vi "DefaultBaseDirectory.vi"(11 "base directory in":path) -> (3 "base directory":path)   [LabVIEW 2017, in "GlobalConfiguration.lvlib"]
uses:
  <vilib>/addons/InsightCM/Utilities/GlobalConfiguration/GlobalConfiguration.lvlib
panel:
  # "Note: Set this before anything else runs"
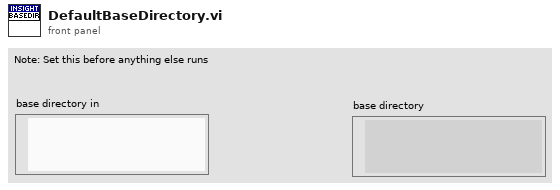
[diagram p1: front panel]
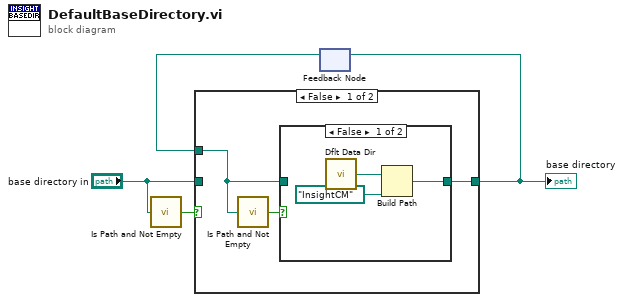
[diagram p0: block diagram]
diagram:
  n1 = call <vilib>:"Is Path and Not Empty.vi"("path"="base directory in") -> ("Is Path and Not Empty?"=w4:bool)  [unwired: 4 in]
  n2 = feedback #1() -> (w2:path)  [unwired: 1 in]
  n3 = case shown="False" w4 {
    tunnel: [w7 w12] -> w1
    tunnel: "base directory in" -> [_ w12]
    tunnel: w2 -> [w5 _]
    frame False {
      n4 = call <vilib>:"Is Path and Not Empty.vi"("path"=w5) -> ("Is Path and Not Empty?"=w6:bool)  [unwired: 4 in]
      n5 = case shown="False" w6 {
        tunnel: [w10 w11] -> w7
        tunnel: w5 -> [_ w11]
        frame False {
          n6 = call <vilib>:"Dflt Data Dir.vi"() -> ("App:Default Data Directory"=w9:path)
          n7 = Build Path(base path=w9, name or relative path=path "InsightCM" ("system directory")) -> (appended path=w10:path)
        }
        frame True {
        }
      }
    }
    frame True {
    }
  }
  "base directory" <- w1
  n8 = feedback-in #1(w1) -> ()
